vi "isViewerRunning.vi"(8 "error in (no error)":errorcluster, 11 "ImageStreamViewer in":refnum<class "ImageStreamViewer.lvclass">) -> (0 "error out":errorcluster, 2 "running?":bool, 3 "ImageStreamViewer out":refnum<class "ImageStreamViewer.lvclass">)   [LabVIEW 2009, in "Views.lvlib" / "Camera.lvlib" / "ImageStreamViewer.lvclass"]
uses:
  ImageStreamViewer.lvclass
  ImageStreamViewer.lvclass/ImageStreamViewer.ctl
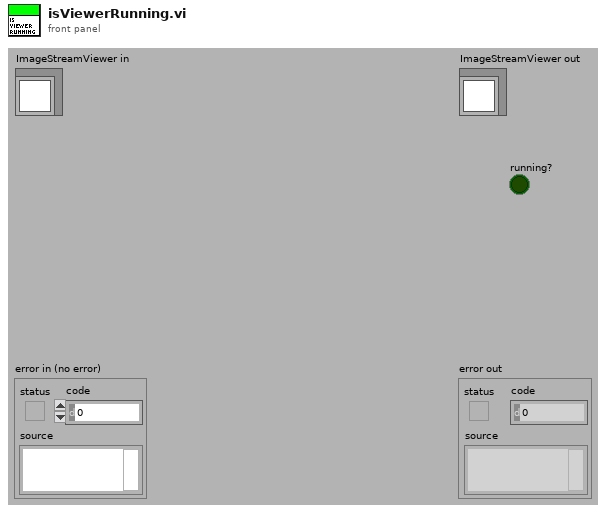
[diagram p1: front panel]
types:
  T1 = enum32{"Bad", "Idle", "Run top level", "Running"}
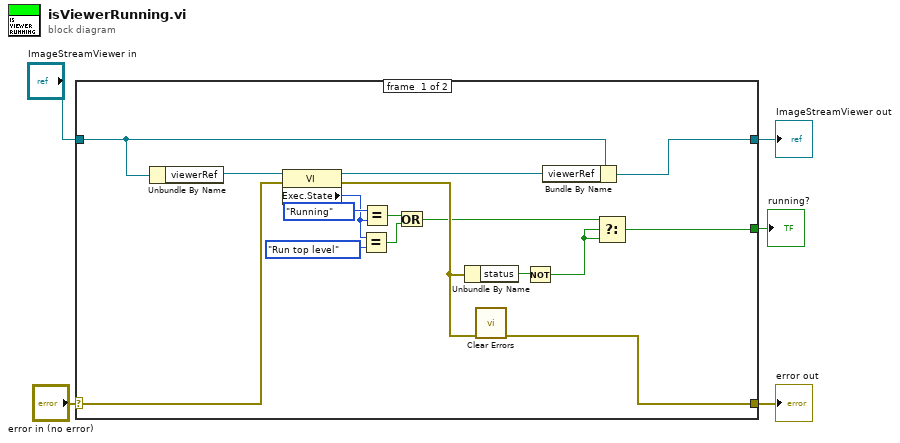
[diagram p0: block diagram]
diagram:
  n1 = case shown="No Error" "error in (no error)" {
    selector: "error in (no error)" -> [w7 w23]
    tunnel: [w8 w23] -> w4
    tunnel: [w9 w22] -> w2
    tunnel: "ImageStreamViewer in" -> [w10 w22]
    tunnel: [w6 _] -> w1
    frame #0 {
      n2 = Unbundle By Name(w10) -> ("viewerRef"=w21:refnum<vi>)
      n3 = property class="VI"(reference=w21, error in=w7) -> (reference out=w18:refnum<vi>, error out=w20:errorcluster, "Exec.State"=w16:T1)
      n4 = Equal?(x=w16, y=T1."Run top level" ("Execution:State")) -> (x = y?=w13:bool)
      n5 = Equal?(x=T1."Running" ("Execution:State"), y=w16) -> (x = y?=w14:bool)
      n6 = Or(x=w14, y=w13) -> (x .or. y?=w12:bool)
      n7 = Unbundle By Name(w20) -> ("status"=w19:bool)
      n8 = call <vilib>:"Clear Errors.vi"("error in (no error)"=w20) -> ("error out"=w8:errorcluster)  [unwired: 6 in]
      n9 = Not(x=w19) -> (.not. x?=w11:bool)
      n10 = Bundle By Name(cluster=w10, "viewerRef"=w18) -> (w9:refnum<class "ImageStreamViewer.lvclass">)
      n11 = Select(t=w12, s=w11, f=w11) -> (s? t:f=w6:bool)
    }
    frame #1 {
    }
  }
  "error out" <- w4
  "ImageStreamViewer out" <- w2
  "running?" <- w1
